vi "LCV Switch Valve To Position.vi"(8 "error in (no error)":errorcluster caption="Fehler (Eingang, kein Fehler)", 10 "Logical Valve Position":i32, 11 "Valve Handle":i64) -> (0 "error out":errorcluster caption="Fehler (Ausgang)")   [LabVIEW 2023, in "labbCAN_Valve_API.lvlib"]
doc: "LCV_Func long LCV_CALL LCV_SwitchValveToPosition(dev_hdl hValve,\n int LogicalValvePosition);"
uses:
  labbCAN_Valve_API.lvlib
  labbCAN_Valve_API.dll
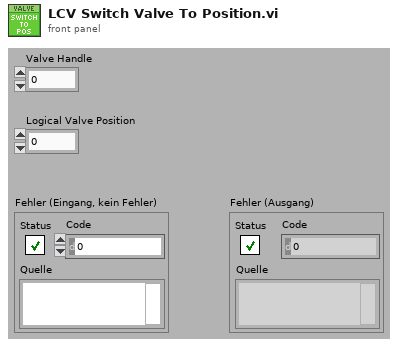
[diagram p1: front panel]
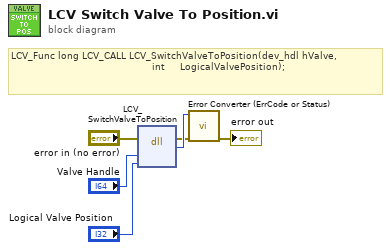
[diagram p0: block diagram]
diagram:
  # "LCV_Func long LCV_CALL LCV_SwitchValveToPosition(dev_hdl hValve,\n\t                                              int     LogicalValvePosition);"
  n1 = dll-call lib="C:/GIT/DensityGradientProject/CETONI_SDK/labbCAN_Valve_API.*" fn="LCV_SwitchValveToPosition"(error in="error in (no error)", "hValve"="Valve Handle", "LogicalValvePosition"="Logical Valve Position") -> (error out=w2:errorcluster, "Rückgabetyp"=w3:i32)  [unwired: 4 in, 1 out]
  n2 = call "Error Converter (ErrCode or Status).vi"("error in (no error)"=w2, "error code"=w3) -> ("error out"=→"error out":errorcluster)  [unwired: 9 in]
